vi "4-2 matrice 3xM - matrice max - matrice 100x sol.vi"() -> ()   [LabVIEW 2012]
panel:
  out "B(i)":dbl[](array[numeric]) format="%.2f"
  out "A(i)":dbl[](array[numeric]) format="%.2f"
  out "c(i)":dbl[](array[numeric]) format="%.2f"
  out "b(i)":dbl[](array[numeric]) format="%.2f"
  out "a(i)":dbl[](array[numeric]) format="%.2f"
  out "Matrice":dbl[][](array[numeric]) format="%.2f"
  in  "Numero di colonne":i32=4
  # "Realizzare, mediante un generatore di numeri casuali,\n una matrice 3xN [a(i), b(i), c(i) con i che varia  da 0 a N-1] con N impostabile da pannello .\n\n Utilizzando la matrice generata dal SubVi precedente, generare due vettori\n  A(i) e B(i)  [0 <= i <= N-1] con A(i) = Max [a(i),b(i)]  e B(i) = 100*[b(i) + c(N-1-i)]"
  # "DOMANDE: \n- nel ciclo for per la creazione di A(i), con l'indicizzazione abilitata in ingresso, \nil programma confronta automaticamente la prima,poi la seconda e infine la terza\nriga del vettore in ingresso, se invece collego l'indice di Array Subset all'indice del \nciclo, il confronto parte la prima volta dall'elemento 0-0, poi dall'elemento 1-1 e poi dal\n2-2 (che non c' quindi viene passato in uscita 0). Perch? Cosa devo cambiare perch \nfunzioni se l'indicizzazione non  abilitata?\n- nella creazione di B(i), ogni tanto la somma delle componenti non  esatta ( inferiore di 1 unit),\nperch? Il fatto che se rappresento le componenti di B(i) come decimali ottengo cifre sgnificative\ndopo la virgola  dovuto solo al fatto che i numeri random sono generati con molte cifre?"
  # "RISPOSTE:\n- per ottenere lo stesso risultato con l'indicizzazione non abilitata devo fare \"add dimension\" su \"array subset\",\ncollegare l'indice i del ciclo al primo indice di array subset e lasciare scollegato il secondo. Se faccio come nel\ntesto della domanda vengono confrontati gli elementi di uno stesso vettore.\n-  dovuto al fatto che i numeri random sono generati con molte cifre decimali, se la parte decimale supera 5\nil risultato viene arrotondato all'intero successivo."
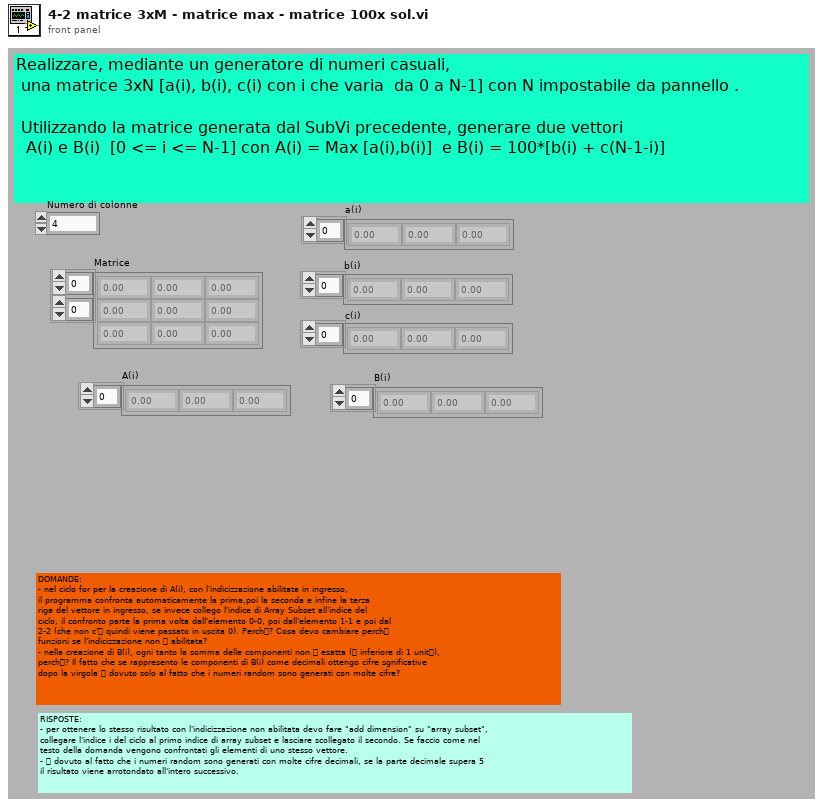
[diagram p1: front panel]
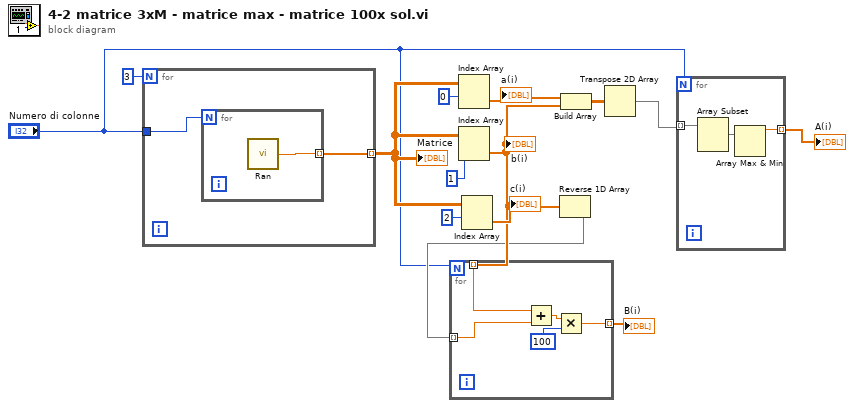
[diagram p0: block diagram]
diagram:
  n1 = for {
    N: 3 -> [_]
    tunnel: "Numero di colonne" -> [w16]
    tunnel: [w15] -> w13 mode=indexing
    n2 = for {
      N: w16 -> [_]
      tunnel: [w17] -> w15 mode=indexing
      n3 = call "Ran.vi"() -> ("out num"=w17:dbl)  [unwired: 5 in]
    }
  }
  "Matrice" <- w13
  n4 = Index Array(array=w13, index (row)=0 ("Array Index")) -> (element=w11:dbl[])  [unwired: 1 in]
  "a(i)" <- w11
  n5 = Index Array(array=w13, index (row)=1 ("Index")) -> (element=w4:dbl[])  [unwired: 1 in]
  "b(i)" <- w4
  n6 = Index Array(array=w13, index (row)=2 ("Index (row)")) -> (element=w10:dbl[])  [unwired: 1 in]
  "c(i)" <- w10
  n7 = Reverse 1D Array(array=w10) -> (reversed array=w3:dbl[])
  n8 = for {
    N: "Numero di colonne" -> [_]
    tunnel: w4 -> [w19] mode=indexing
    tunnel: w3 -> [w18] mode=indexing
    tunnel: [w20] -> w2 mode=indexing
    n9 = Add(x=w19, y=w18) -> (x+y=w22:dbl)
    n10 = Multiply(x=w22, y=100) -> (x*y=w20:dbl)
  }
  "B(i)" <- w2
  n11 = Build Array(w11, w4) -> (w5:dbl[][])
  n12 = Transpose 2D Array(2D array=w5) -> (transposed array=w6:dbl[][])
  n13 = for {
    N: "Numero di colonne" -> [_]
    tunnel: [w25] -> w7 mode=indexing
    tunnel: w6 -> [w24] mode=indexing
    n14 = Array Subset(array=w24) -> (w23:dbl[])  [unwired: 2 in]
    n15 = Array Max & Min(array=w23) -> (max value=w25:dbl)  [unwired: 3 out]
  }
  "A(i)" <- w7
